vi "Add Overlay Meta Fields.vi"(8 "error in (no error)":errorcluster, 10 "Meta Fields":string[](array[string]), 11 "Config Storage in":refnum<class "Config Storage.lvclass">) -> (0 "error out":errorcluster, 3 "Config Storage out":refnum<class "Config Storage.lvclass">)   [LabVIEW 2020, in "CDM-Config.lvlib" / "Config Storage.lvclass"]
uses:
  Config Storage.lvclass
  Config Storage.lvclass/Config Storage.ctl
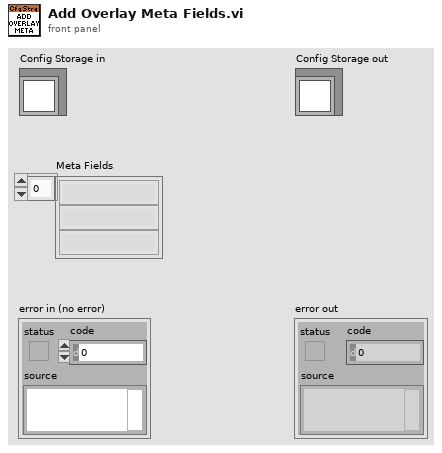
[diagram p1: front panel]
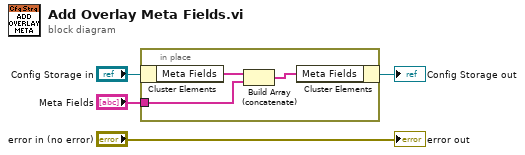
[diagram p0: block diagram]
diagram:
  n1 = in-place {
    in-place-border: "Meta Fields" -> [w6]
    n2 = in-place-cluster #1("Config Storage in") -> ("Meta Fields"=w7:string[])
    n3 = Build Array (concatenate)(w7, w6) -> (w5:string[])
    n4 = in-place-cluster #1("Meta Fields"=w5) -> (→"Config Storage out":refnum<class "Config Storage.lvclass">)
  }
  "error out" <- "error in (no error)"
